vi "CardStringtoArray.vi"(3 "error in (no error)":errorcluster, 5 "Card In":string) -> (0 "error out":errorcluster, 1 "N:r Cards":i32, 2 "Card Array":string[](array[string]))   [LabVIEW 2011]
doc: "The vi are transforming the card string to an array."
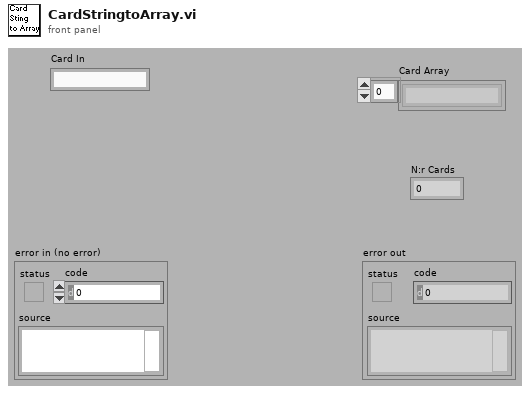
[diagram p1: front panel]
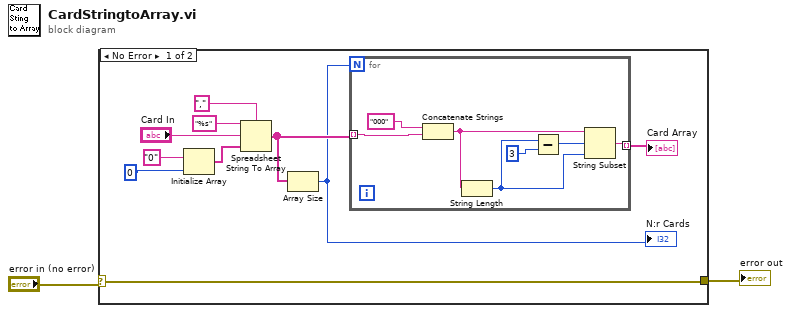
[diagram p0: block diagram]
diagram:
  n1 = case shown="No Error" "error in (no error)" {
    selector: "error in (no error)" -> [w7 w20]
    tunnel: [w7 w20] -> w1
    frame No Error {
      n2 = Initialize Array("0", 0) -> (w3:string[])
      n3 = Spreadsheet String To Array(delimiter (Tab)=",", format string="%s", spreadsheet string="Card In", array type (2D Dbl)=w3) -> (array=w6:string[])
      n4 = Array Size(array=w6) -> (size(s)=w4:i32)
      "N:r Cards" <- w4
      n5 = for {
        N: w4 -> [_]
        tunnel: w6 -> [w13] mode=indexing
        tunnel: [w14] -> w5 mode=indexing
        n6 = Concatenate Strings("000", w13) -> (w18:string)
        n7 = String Length(string=w18) -> (length=w15:i32)
        n8 = Subtract(x=w15, y=3) -> (x-y=w17:i32)
        n9 = String Subset(string=w18, offset (0)=w17, length (rest)=w15) -> (substring=w14:string)
      }
      "Card Array" <- w5
    }
    frame Error {
    }
  }
  "error out" <- w1
